vi "Read SubComponent Data - Raw.vi"(8 "error in (no error)":errorcluster, 11 "Bus Monitor in":refnum<class "Bus Monitor.lvclass">) -> (0 "error out":errorcluster, 1 "Raw Data":u64[](array[numeric]), 2 "Parameter":string[](array[string]), 3 "Bus Monitor out":refnum<class "Bus Monitor.lvclass">)   [LabVIEW 2020, in "BCI-1553 API.lvlib" / "Bus Monitor.lvclass"]
doc: "Reads the raw data values transacted for each filter parameters for the Bus Monitor."
uses:
  Bus Monitor.lvclass
  Bus Monitor.lvclass/Bus Monitor.ctl
  Dependencies/Registry/Registry.lvclass/Registry.ctl
  Filters/Filter/Filter.lvclass
  Dependencies/Registry/Registry.lvclass
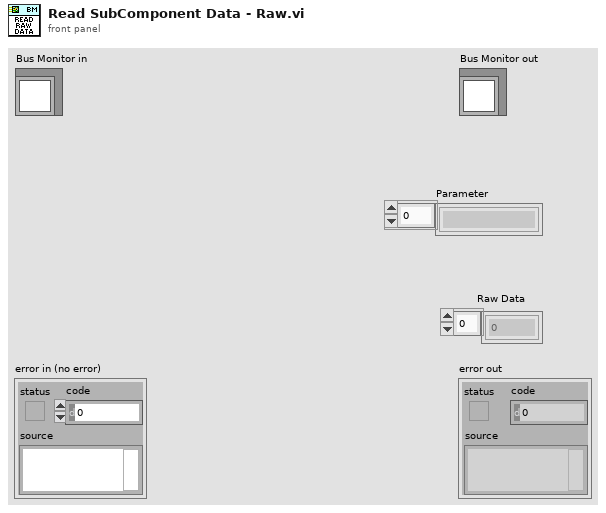
[diagram p1: front panel]
types:
  T1 = typedef "BCI-1553 API.lvlib/Parameter Table Data.ctl" = cluster{"Parameter Name":string, "Base Word":u16, "Address":u16, "Value":u64, "Mask":u16[], "Scaling Info":T2}
  T2 = typedef "BCI-1553 API.lvlib/Scaling Information.ctl" = cluster{"Bit Offset":i32, "Bit Count":i32, "LSB Resolution":dbl, "2's Complement":bool, "Big Endian":bool, "Sign Bit":bool}
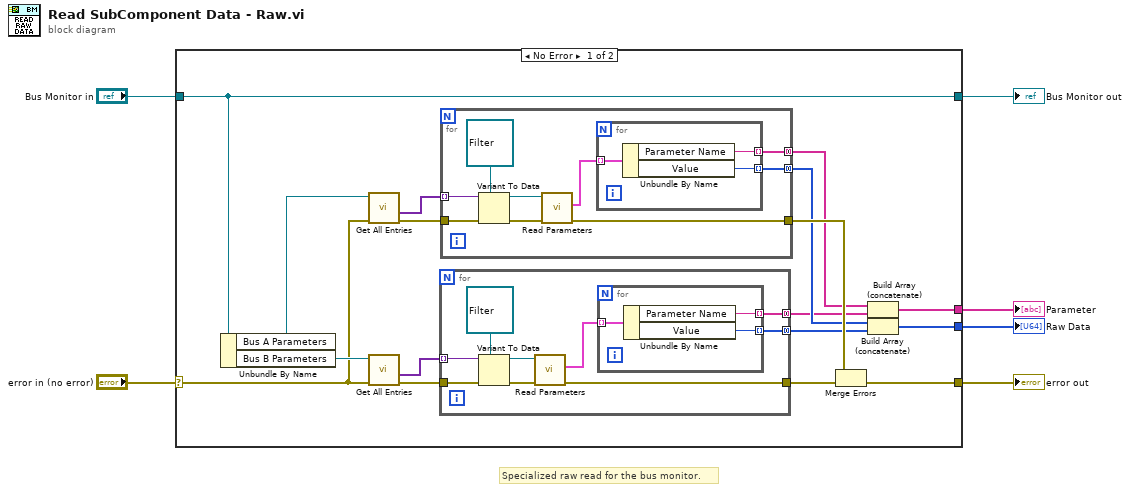
[diagram p0: block diagram]
diagram:
  # "Specialized raw read for the bus monitor."
  n1 = case shown="No Error" "error in (no error)" {
    selector: "error in (no error)" -> [w8 w48]
    tunnel: "Bus Monitor in" -> [w7 w49]
    tunnel: [w15 w48] -> w5
    tunnel: [w10 _] -> w4
    tunnel: [w9 _] -> w3
    tunnel: [w7 w49] -> w1
    frame No Error {
      n2 = Unbundle By Name(w7) -> ("Bus A Parameters"=w23:refnum<class "Registry.lvclass">, "Bus B Parameters"=w22:refnum<class "Registry.lvclass">)
      n3 = call "Get All Entries.vi"("error in (no error)"=w8, "Registry in"=w23) -> ("error out"=w18:errorcluster, "Values"=w20:variant[])  [unwired: 7 in, 1 out]
      n4 = call "Get All Entries.vi"("error in (no error)"=w8, "Registry in"=w22) -> ("error out"=w19:errorcluster, "Values"=w21:variant[])  [unwired: 7 in, 1 out]
      n5 = for {
        tunnel: w21 -> [w44] mode=indexing
        tunnel: w19 -> [w43]
        tunnel: [w39] -> w17
        tunnel: [w37] -> w12 mode=concatenating
        tunnel: [w36] -> w14 mode=concatenating
        n6 = Variant To Data(error in=w43, type=refnum<class "Filter.lvclass"> refnum ("SLSC 1553 API.lvlib:Filter.lvclass"), Variant=w44) -> (data=w41:refnum<class "Filter.lvclass">, error out=w40:errorcluster)
        n7 = call-dynamic "Read Parameters.vi"("error in (no error)"=w40, "Filter in"=w41) -> ("error out"=w39:errorcluster, "Parameters"=w38:T1[])  [unwired: 7 in, 1 out]
        n8 = for {
          tunnel: w38 -> [w47] mode=indexing
          tunnel: [w46] -> w37 mode=indexing
          tunnel: [w45] -> w36 mode=indexing
          n9 = Unbundle By Name(w47) -> ("Parameter Name"=w46:string, "Value"=w45:u64)
        }
      }
      n10 = for {
        tunnel: w20 -> [w31] mode=indexing
        tunnel: w18 -> [w32]
        tunnel: [w27] -> w16
        tunnel: [w25] -> w11 mode=concatenating
        tunnel: [w24] -> w13 mode=concatenating
        n11 = Variant To Data(error in=w32, type=refnum<class "Filter.lvclass"> refnum ("SLSC 1553 API.lvlib:Filter.lvclass"), Variant=w31) -> (data=w29:refnum<class "Filter.lvclass">, error out=w28:errorcluster)
        n12 = call-dynamic "Read Parameters.vi"("error in (no error)"=w28, "Filter in"=w29) -> ("error out"=w27:errorcluster, "Parameters"=w26:T1[])  [unwired: 7 in, 1 out]
        n13 = for {
          tunnel: [w35] -> w25 mode=indexing
          tunnel: [w34] -> w24 mode=indexing
          tunnel: w26 -> [w33] mode=indexing
          n14 = Unbundle By Name(w33) -> ("Parameter Name"=w35:string, "Value"=w34:u64)
        }
      }
      n15 = Merge Errors(w16, w17) -> (w15:errorcluster)
      n16 = Build Array (concatenate)(w11, w12) -> (w10:string[])
      n17 = Build Array (concatenate)(w13, w14) -> (w9:u64[])
    }
    frame Error {
    }
  }
  "error out" <- w5
  "Bus Monitor out" <- w1
  "Raw Data" <- w3
  "Parameter" <- w4
